vi "Override State.vi"(6 "Raw Pressure":dbl=nan, 7 "Delivery Occurence":refnum<k4>, 8 "error in (no error)":errorcluster, 9 "Pressure":dbl=nan, 10 "State":T1, 11 "cRIO Vacuum in":refnum<class "cRIO Vacuum.lvclass">) -> (0 "error out":errorcluster, 3 "cRIO Vacuum out":refnum<class "cRIO Vacuum.lvclass">)   [LabVIEW 2015, in "cRIO-Carbondioxide.lvlib" / "CO2-Actor.lvlib" / "cRIO Vacuum.lvclass"]
uses:
  cRIO Vacuum.lvclass
  Controls/Vacuum State Enumerator.ctl
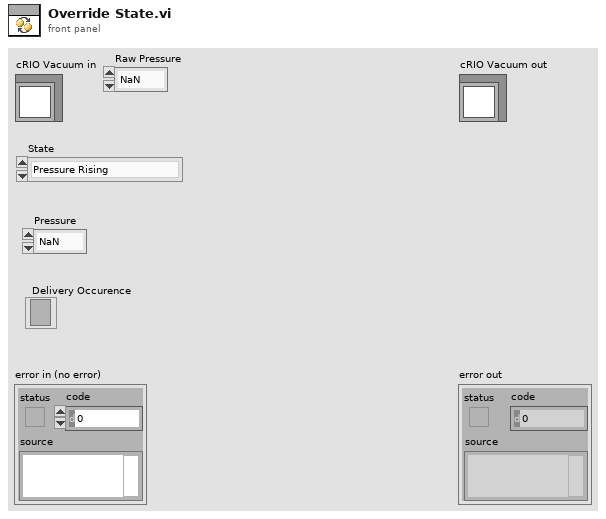
[diagram p1: front panel]
types:
  T1 = typedef "Vacuum State Enumerator.ctl" = enum16{"Pressure Rising", "Plateau", "Pressure Dropping", "Valley", "Low Valley", "Leak", "Unknown"}
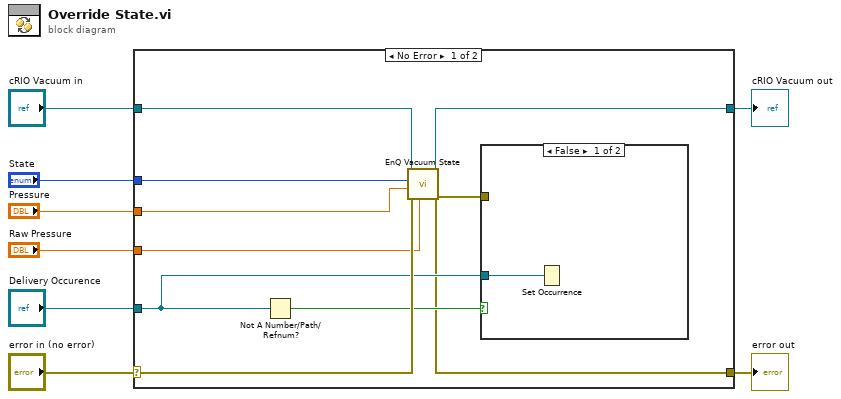
[diagram p0: block diagram]
diagram:
  n1 = case shown="No Error" "error in (no error)" {
    selector: "error in (no error)" -> [w15 w20]
    tunnel: [w10 w20] -> w7
    tunnel: [w16 w19] -> w5
    tunnel: "cRIO Vacuum in" -> [w17 w19]
    tunnel: "State" -> [w14 _]
    tunnel: "Pressure" -> [w13 _]
    tunnel: "Delivery Occurence" -> [w11 _]
    tunnel: "Raw Pressure" -> [w9 _]
    frame No Error {
      n2 = Not A Number/Path/Refnum?(number/path/refnum=w11) -> (NaN/Path/Refnum?=w12:bool)
      n3 = call "EnQ Vacuum State.vi"("Raw Pressure"=w9, "error in (no error)"=w15, "Pressure"=w13, "State"=w14, "cRIO Vacuum in"=w17) -> ("error out"=w10:errorcluster, "cRIO Vacuum out"=w16:refnum<class "cRIO Vacuum.lvclass">)  [unwired: 1 in, 4 out]
      n4 = case shown="False" w12 {
        tunnel: w11 -> [w18 _]
        tunnel: w10 -> [_ _]
        frame False {
          n5 = Set Occurrence(w18) -> ()
        }
        frame True {
        }
      }
    }
    frame Error {
    }
  }
  "error out" <- w7
  "cRIO Vacuum out" <- w5
